vi "Therapy&Scan.vi"(7 "VISA session in":refnum<visa-resource-name>, 8 "File Name In":string, 9 "Motion Settings":T1={"No Motion?"=FALSE, "Motion System"=enum."NI 735x", "Motion Bd ID"=1, "Motion Profile"="SMAC1", "# Axis"=1, "Reverse Z axis?"=TRUE, "SMAC Axis"=0, "scan pair"=enum."y-(x) scan", "RT fps"=6.0, "Steps per mm"=[1000, 1000, 1000, 1000], "Motor Parameters"={"velocity ct/s"=[10000.0, 10000.0, 10000.0, 50000.0], "accel ct/s^2"=[50000.0, 50000.0, 50000.0, 200000.0]}, "One Way Scan"=FALSE, "Reverse One Way Scan"=FALSE, "Global Position (mm)"=[], "Plane"=0, "Distance between\nscan lines (um)"=0.0, "Distance between\nscan planes (um)"=0.0, "number of scan planes"=1, "Total steps in line"=0, "Xtra plane\ndistance  (um)"=100, "Xtra planes "=1, "Add Axis"=FALSE, "overshoot cts"=200, "BKPT Shift"=0, "Scan Start Time (ms)"=0, "ESP VISA"="GPIB::1::INSTR", "3rd Axis"=1, "GL Ref Out"=refnum, "Galil Address"=""} {"3rd Axis" items=["x", "y", "z", "w"]; "Xtra planes" min=1; "Xtra plane\ndistance  (um)" min=0; "Distance between\nscan planes (um)" format="%.2f"; "Distance between\nscan lines (um)" format="%.2f"; "SMAC Axis" items=["None"=0, "Axis 1"=1, "Axis 2"=2, "Axis 3"=3, "Axis 4"=4, "Axis 5"=5, "Axis 6"=6, "Axis 7"=7, "Axis 8"=8, "Vector Space 1"=17, "Vector Space 2"=18, "Vector Space 3"=19, "Vector Space 4"=20]; "Motion Bd ID" min=1 max=32 step=1}, 10 "Therapy Parameters":T10={"Theraputic Freq (MHz)"=1.0, "Time on"=0.0, "Therapy amplitude (mV)"=50.0, "Lines Before"=0, "Lines After"=0} {"Therapy amplitude (mV)" format="%.2f"; "Time on" format="%.2f"; "Theraputic Freq (MHz)" format="%.2f"}, 11 "Digitizer Settings":T5={"Digitizer delay (us) "=0.0, "rf points per line"=2048, "lines per plane"=128, "Samp Rate (Hz)"=100000000.0, "Additional dig delay (us)"=0.0, "Voltage Scale"=0.4, "Pre-Looks"=0, "Offset delay (us)"=0.0, "bits A/D"=8, "Avg Num"=1, "DigTimeOut"=5.0, "Rel Dig Delay"=0.0, "Dig Ch"=0, "LeCroyCluster"={"LeCroy Channels"=[TRUE, FALSE, FALSE, FALSE], "LC read pt offset"=0.0, "Sweep Avg"=FALSE}, "Main Digitizer"=enum."NI Digitizer", "Dig Config"=enum."Single channel", "Digitizer ID Cluster"={"Acqiris/Alazar/SP ID"=[], "NI Instr Handles"=[], "LeCroy VISA"="", "GaGe Handle"={"Handle"=0, "Sample size"=0, "Resolution"=0, "Offset"=0, "Channels"=0, "Boards"=0}, "ATS Ref"="ATS9350", "Acqiris Address"=["PCI::INSTR0"], "ADQRef"=refnum, "adq_cu_ptr"=refnum}, "Trigger Settings"={"Trig Source"=1, "Trig Coupling"=0, "Trig Slope"=0, "Level (mV)"=1500.0}, "Bulk Acq"=FALSE, "Bulk Start Indexes"=[], "Data Ref RF"=refnum, "NI ID/Channel"=[], "Total Dig CH"=1, "Xtra Ann Trig delay (us)"=10.0, "Fix Z Delay?"=FALSE, "One Way Transmission?"=FALSE, "Data Ref Log"=refnum} {"Trigger Settings"."Trig Slope" items=["Positive", "Negative"]; "Trigger Settings"."Level (mV)" format="%.2f"; "Trigger Settings"."Trig Coupling" items=["DC 1 MOhm", "AC 1 MOhm", "DC 50 Ohm", "AC 50 Ohm"]; "Trigger Settings"."Trig Source" items=["Chan 1", "External"]; "Rel Dig Delay" format="%.2f"; "DigTimeOut" format="%.2f"; "Avg Num" min=1; "Offset delay (us)" format="%.2f"; "Additional dig delay (us)" format="%.2f"; "Digitizer delay (us)" format="%.2f"}) -> (0 "Error Message":string, 1 "Scan Data":i16[][](array[numeric]), 2 "Scan Params":T9={"File Name"="", "Keep?"=FALSE, "Synth Foc?"=TRUE, "Microscopy Scan Mode"=enum."Overview Scan"})   [LabVIEW 2022 SP3]
uses:
  Controls/ScanParams.ctl
  Digitizers/-DigitizerRoutines/DigitizerSettings.ctl
  Digitizers/-DigitizerRoutines/Digitizer.ctl
  Digitizers/-DigitizerRoutines/DigConfig.ctl
  Digitizers/-DigitizerRoutines/DigitizerID.ctl
  C:/Windows/System32/ADQAPI_dotNet_helper.dll
  Motion Controllers/NI_controller/-NI_MotionRoutines/MotionParameters.ctl
  Motion Controllers/NI_controller/-NI_MotionRoutines/MotionSys.ctl
  Motion Controllers/-MotionRoutines/ScanAxis.ctl
  Motion Controllers/-MotionRoutines/3rdAxis.ctl
  Motion Controllers/-MotionRoutines/MotionGlobals.vi
  <vilib>/DAQmx/create/channels.llb/DAQmx Create Channel (CO-Pulse Generation-Time).vi
panel:
  # "1-D and 2-D B scan settings"
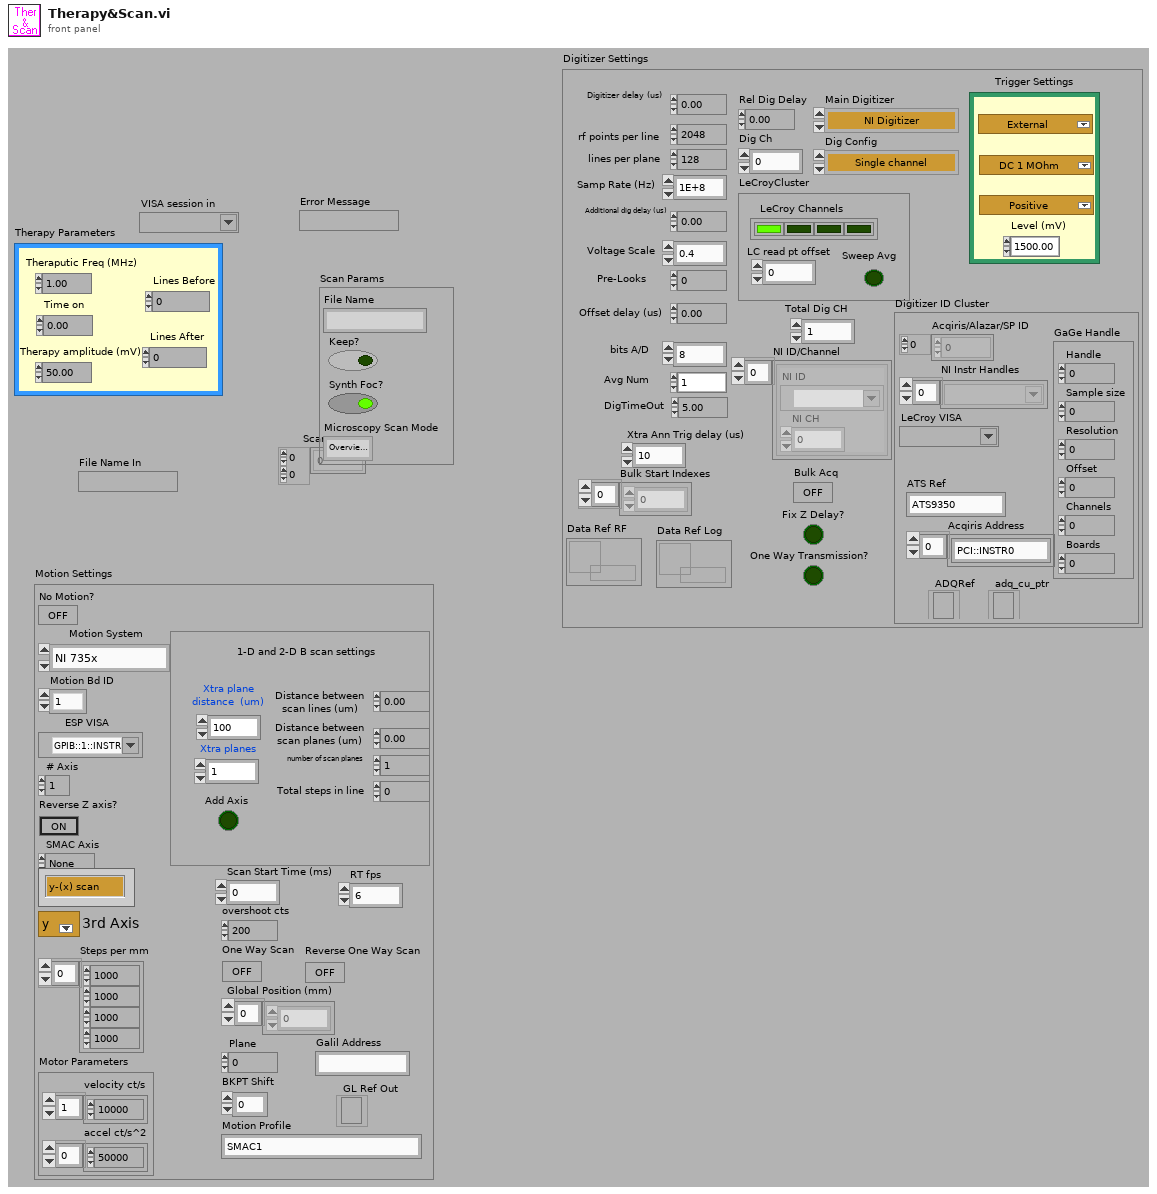
[diagram p1: front panel]
types:
  T1 = typedef "MotionParameters.ctl" = cluster{"No Motion?":bool, "Motion System":T2, "Motion Bd ID":u8, "Motion Profile":string, "# Axis":i8, "Reverse Z axis?":bool, "SMAC Axis":u16, "scan pair":T3, "RT fps":sgl, "Steps per mm":i32[], "Motor Parameters":cluster{"velocity ct/s":dbl[], "accel ct/s^2":dbl[]}, "One Way Scan":bool, "Reverse One Way Scan":bool, "Global Position (mm)":dbl[], "Plane":i32, "Distance between\nscan lines (um)":sgl, "Distance between\nscan planes (um)":sgl, "number of scan planes":i32, "Total steps in line":i32, "Xtra plane\ndistance  (um)":i32, "Xtra planes ":i32, "Add Axis":bool, "overshoot cts":i32, "BKPT Shift":i32, "Scan Start Time (ms)":u32, "ESP VISA":refnum<visa-resource-name>, "3rd Axis":T4, "GL Ref Out":refnum<k7>, "Galil Address":string}
  T2 = typedef "MotionSys.ctl" = enum16{"MM3000", "NI 735x", "Newport ESP", "No Motion Card", "Galil"}
  T3 = typedef "ScanAxis.ctl" = enum16{"y-(x) scan", "x-(y) scan", "z-(x) scan", "z-(y) scan", "y-(z) scan", "x-(z) scan", "w-(x) scan", "w-(y) scan", "w-(z) scan", "x-(w) scan", "y-(w) scan", "z-(w) scan"}
  T4 = typedef "3rdAxis.ctl" = u16
  T5 = typedef "DigitizerSettings.ctl" = cluster{"Digitizer delay (us) ":dbl, "rf points per line":i32, "lines per plane":i32, "Samp Rate (Hz)":dbl, "Additional dig delay (us)":dbl, "Voltage Scale":dbl, "Pre-Looks":i32, "Offset delay (us)":dbl, "bits A/D":i8, "Avg Num":i32, "DigTimeOut":sgl, "Rel Dig Delay":sgl, "Dig Ch":i32, "LeCroyCluster":cluster{"LeCroy Channels":bool[], "LC read pt offset":dbl, "Sweep Avg":bool}, "Main Digitizer":T6, "Dig Config":T7, "Digitizer ID Cluster":T8, "Trigger Settings":cluster{"Trig Source":u16, "Trig Coupling":u16, "Trig Slope":u16, "Level (mV)":dbl}, "Bulk Acq":bool, "Bulk Start Indexes":i32[], "Data Ref RF":refnum<data-value>, "NI ID/Channel":cluster{"NI ID":refnum<k15>, "NI CH":i32}[], "Total Dig CH":i32, "Xtra Ann Trig delay (us)":dbl, "Fix Z Delay?":bool, "One Way Transmission?":bool, "Data Ref Log":refnum<data-value>}
  T6 = typedef "Digitizer.ctl" = enum16{"Acqiris Digitizer", "NI Digitizer", "LeCroy", "GaGe", "AlazarTech", "No Digitizer", "Teledyne"}
  T7 = typedef "DigConfig.ctl" = enum16{"Single channel", "2 Chans w/ 2 Acqiris", "2 Chans w/ 1 Acqiris", "5-CH Pulser New", "5-CH pulser w/ ann array", "5-pass style ann array", "Empty"}
  T8 = typedef "DigitizerID.ctl" = cluster{"Acqiris/Alazar/SP ID":u32[], "NI Instr Handles":refnum<k15>[], "LeCroy VISA":refnum<visa-resource-name>, "GaGe Handle":cluster{"Handle":u32, "Sample size":u32, "Resolution":i32, "Offset":i32, "Channels":u32, "Boards":u32}, "ATS Ref":string, "Acqiris Address":string[], "ADQRef":refnum<k24>, "adq_cu_ptr":refnum<k24>}
  T9 = typedef "ScanParams.ctl" = cluster{"File Name":string, "Keep?":bool, "Synth Foc?":bool, "Microscopy Scan Mode":enum32{"Level X", "Level Y", "Overview Scan", "Detailed Scan", "V-Z Scan"}}
  T10 = cluster{"Theraputic Freq (MHz)":dbl, "Time on":dbl, "Therapy amplitude (mV)":dbl, "Lines Before":i16, "Lines After":i16}
  T11 = enum32{"Level X", "Level Y", "Overview Scan", "Detailed Scan", "V-Z Scan"}
  T12 = cluster{i32, "Theraputic Freq (MHz)":dbl, "Therapy amplitude (mV)":dbl}
  T13 = cluster{sgl, "Gain [dB]  ":sgl, "Atten (dB)":sgl}
  T14 = cluster{"File Name In":string, bool, bool, "Microscopy Scan Mode":enum32{"Level X", "Level Y", "Overview Scan", "Detailed Scan", "V-Z Scan"}}
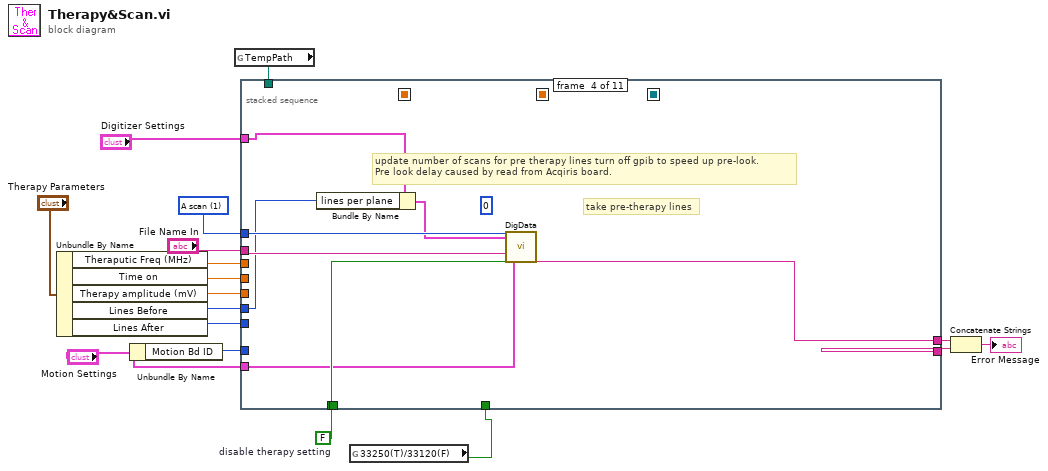
[diagram p0: block diagram]
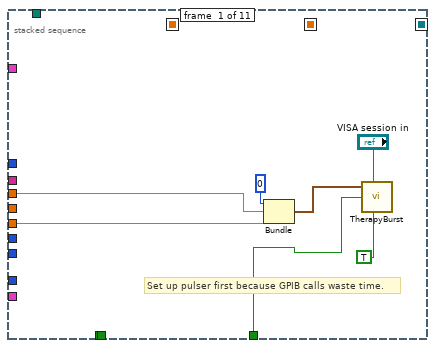
[diagram p2: hidden frame]
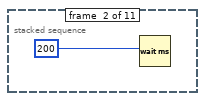
[diagram p3: hidden frame]
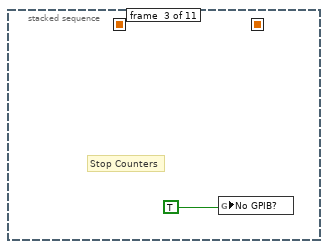
[diagram p4: hidden frame]
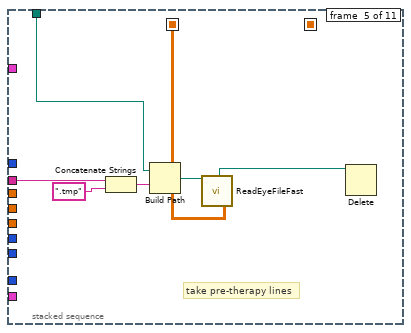
[diagram p5: hidden frame]
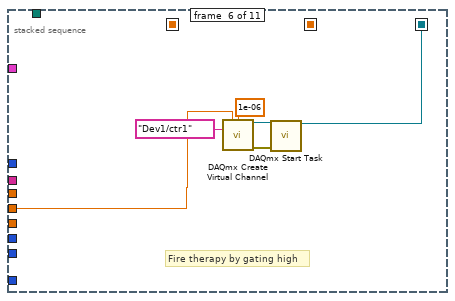
[diagram p6: hidden frame]
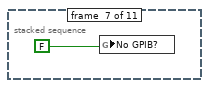
[diagram p7: hidden frame]
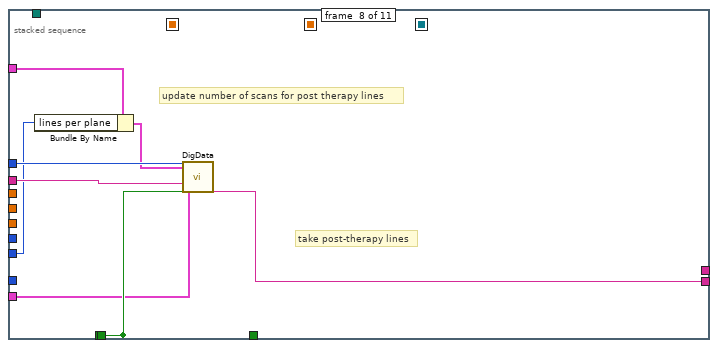
[diagram p8: hidden frame]
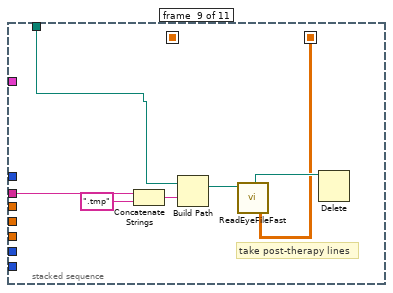
[diagram p9: hidden frame]
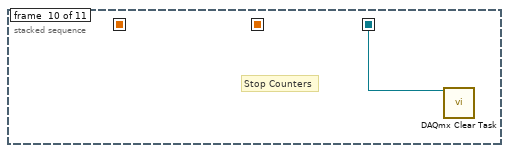
[diagram p10: hidden frame]
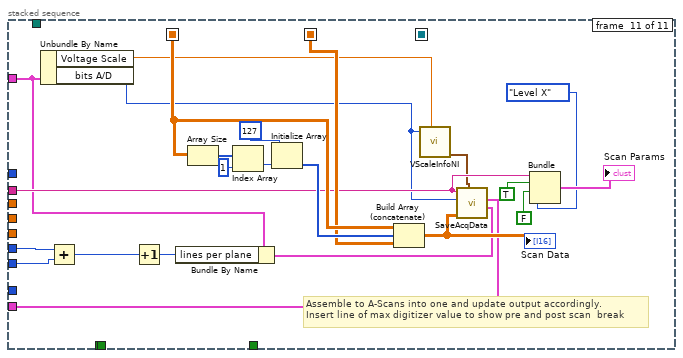
[diagram p11: hidden frame]
diagram:
  w12 = u16 1 items=["Therapy", "A scan", "A scan w/ therapy", "1-D B Scan", "1-D B Scan w/ Therapy", "2-D B Scan", "2-D B Scan w/ Therapy"] ("Type of scan")
  w13 = FALSE  # disable therapy setting
  n1 = Unbundle By Name("Therapy Parameters") -> ("Theraputic Freq (MHz)"=w17:dbl, "Time on"=w16:dbl, "Therapy amplitude (mV)"=w15:dbl, "Lines Before"=w11:i16, "Lines After"=w10:i16)
  n2 = Unbundle By Name("Motion Settings") -> ("Motion Bd ID"=w2:u8)
  n3 = global read "MotionGlobals.vi" "TempPath"() -> (w5:path)
  n4 = global read "MotionGlobals.vi" "33250(T)/33120(F)"() -> (w3:bool)
  n5 = stacked-sequence {
    seq-local: [_ _ _ _ w36 _ _ _ _ _ _] -> [_ _ _ _ _ _ _ _ _ _ w82]
    seq-local: [_ _ _ _ _ _ _ _ w58 _ _] -> [_ _ _ _ _ _ _ _ _ _ w81]
    seq-local: [_ _ _ _ _ w46 _ _ _ _ _] -> [_ _ _ _ _ _ _ _ _ w64 _]
    tunnel: w17 -> [w24 _ _ _ _ _ _ _ _ _ _]
    tunnel: w16 -> [_ _ _ _ _ w47 _ _ _ _ _]
    tunnel: w15 -> [w23 _ _ _ _ _ _ _ _ _ _]
    tunnel: "File Name In" -> [_ _ _ w31 w39 _ _ w54 w61 _ w77]
    tunnel: w13 -> [_ _ _ w34 _ _ _ w53 _ _ _]
    tunnel: w12 -> [_ _ _ w33 _ _ _ w56 _ _ _]
    tunnel: w11 -> [_ _ _ w29 _ _ _ _ _ _ w73]
    tunnel: w10 -> [_ _ _ _ _ _ _ w51 _ _ w72]
    tunnel: [_ _ _ _ _ _ _ w55 _ _ _] -> w9
    tunnel: [_ _ _ w32 _ _ _ _ _ _ _] -> w8
    tunnel: w2 -> [_ _ _ _ _ _ _ _ _ _ _]
    tunnel: w5 -> [_ _ _ _ w35 _ _ _ w57 _ _]
    tunnel: "Digitizer Settings" -> [_ _ _ w30 _ _ _ w52 _ _ w71]
    tunnel: [_ _ _ _ _ _ _ w53 _ _ _] -> _
    tunnel: w3 -> [w18 _ _ _ _ _ _ _ _ _ _]
    tunnel: "Motion Settings" -> [_ _ _ w27 _ _ _ w49 _ _ w69]
    frame #0 {
      # "Set up pulser first because GPIB calls waste time."
      n6 = Bundle(0, "Theraputic Freq (MHz)"=w24, "Therapy amplitude (mV)"=w23) -> (w22:T12)  [unwired: 1 out]
      n7 = call "TherapyBurst.vi"("Input Cluster"=w22, "VISA session in"="VISA session in", "33250(T)/33120(F)"=w18, "Trigger (F) Gate(T)"=TRUE) -> ()  [unwired: 2 in, 3 out]
    }
    frame #1 {
      n8 = Wait (ms)(milliseconds to wait=200) -> ()  [unwired: 1 out]
    }
    frame #2 {
      # "Stop Counters"
      n9 = global write "MotionGlobals.vi" "No GPIB?"(TRUE) -> ()
    }
    frame #3 {
      (unwired) 0 ("BKPT Shift")
      # "update number of scans for pre therapy lines turn off gpib to speed up pre-look.\nPre look delay caused by read from Acqiris board."
      # "take pre-therapy lines"
      n10 = Bundle By Name(cluster=w30, "lines per plane"=w29) -> (w28:T5)
      n11 = call "DigData.vi"("Type of scan"=w33, "Digitizer Settings"=w28, "File Name In"=w31, "Therapy (T)"=w34, "Motion Settings In"=w27) -> ("Error Message"=w32:string)  [unwired: 6 in, 16 out]
    }
    frame #4 {
      # "take pre-therapy lines"
      n12 = Concatenate Strings(w39, ".tmp") -> (w40:string)
      n13 = Build Path(base path=w35, name or relative path=w40) -> (appended path=w37:path)
      n14 = call "ReadEyeFileFast.vi"("new file path"=w37) -> ("new path out"=w38:path, "2-D data array"=w36:sgl[][])  [unwired: 1 in, 16 out]
      n15 = Delete(path (use dialog)=w38) -> ()  [unwired: 1 in, 6 out]
    }
    frame #5 {
      # "Fire therapy by gating high"
      n16 = call-poly <vilib>:"DAQmx Create Virtual Channel.vi"("high time"=w47, "low time"=1e-06, "counter"=tag "Dev1/ctr1") -> ("task out"=w44:refnum<k21>, "error out"=w43:errorcluster)  [unwired: 6 in, 5 out]
      n17 = call <vilib>:"DAQmx Start Task.vi"("task/channels in"=w44, "error in"=w43) -> ("task out"=w46:refnum<k21>)  [unwired: 13 out]
    }
    frame #6 {
      n18 = global write "MotionGlobals.vi" "No GPIB?"(FALSE) -> ()
    }
    frame #7 {
      # "update number of scans for post therapy lines"
      # "take post-therapy lines"
      n19 = Bundle By Name(cluster=w52, "lines per plane"=w51) -> (w50:T5)
      n20 = call "DigData.vi"("Type of scan"=w56, "Digitizer Settings"=w50, "File Name In"=w54, "Therapy (T)"=w53, "Motion Settings In"=w49) -> ("Error Message"=w55:string)  [unwired: 6 in, 16 out]
    }
    frame #8 {
      # "take post-therapy lines"
      n21 = Concatenate Strings(w61, ".tmp") -> (w62:string)
      n22 = Build Path(base path=w57, name or relative path=w62) -> (appended path=w60:path)
      n23 = call "ReadEyeFileFast.vi"("new file path"=w60) -> ("new path out"=w59:path, "2-D data array"=w58:sgl[][])  [unwired: 1 in, 16 out]
      n24 = Delete(path (use dialog)=w59) -> ()  [unwired: 1 in, 6 out]
    }
    frame #9 {
      # "Stop Counters"
      n25 = call <vilib>:"DAQmx Clear Task.vi"("task in"=w64) -> ()  [unwired: 1 in, 14 out]
    }
    frame #10 {
      # "Assemble to A-Scans into one and update output accordingly.\nInsert line of max digitizer value to show pre and post scan  break"
      n26 = Unbundle By Name(w71) -> ("Voltage Scale"=w67:dbl, "bits A/D"=w68:i8)
      n27 = Add(x=w73, y=w72) -> (x+y=w75:i16)
      n28 = Increment(x=w75) -> (x+1=w74:i16)
      n29 = Bundle By Name(cluster=w71, "lines per plane"=w74) -> (w70:T5)
      n30 = Array Size(array=w82) -> (size(s)=w84:i32[])
      n31 = Index Array(array=w84, index=1 ("Index")) -> (element=w83:i32)
      n32 = Initialize Array(i16 127, w83) -> (w86:i16[])
      n33 = Build Array (concatenate)(w82, w86, w81) -> (w80:sgl[][])
      "Scan Data" <- w80
      n34 = call "VScaleInfoNI.vi"("A/D bits"=w68, "gain"=w67) -> ("Voltage Scale"=w66:T13)  [unwired: 5 in, 3 out]
      n35 = call "SaveAcqData.vi"("Digitizer Settings"=w70, "Motion Settings"=w69, "Votage scaling"=w66, "Array"=w80, "Dig Word Size"=w68, "File Name"=w77) -> ()  [unwired: 5 in]
      n36 = Bundle("File Name In"=w77, TRUE, FALSE, "Microscopy Scan Mode"=T11."Level X") -> (→"Scan Params":T14)  [unwired: 1 out]
    }
  }
  n37 = Concatenate Strings(w8, w9) -> (→"Error Message":string)
